vi "ysi.vi"(7 "Initialize":bool, 10 "Time Out (secs)":i32, 11 "YSI Com Port":i32) -> (0 "pH":dbl format="%.2f", 1 "Temperature":dbl format="%.2f", 2 "dis O2":dbl format="%.2f", 3 "ORP":dbl format="%.2f", 4 "spec K":dbl format="%.2f", 5 "Fresh Data":bool, 6 "Time out occurred":bool)   [LabVIEW 2016]
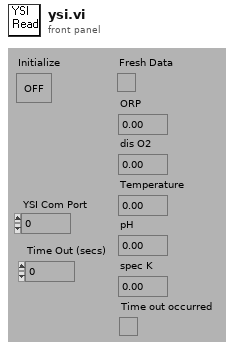
[diagram p1: front panel]
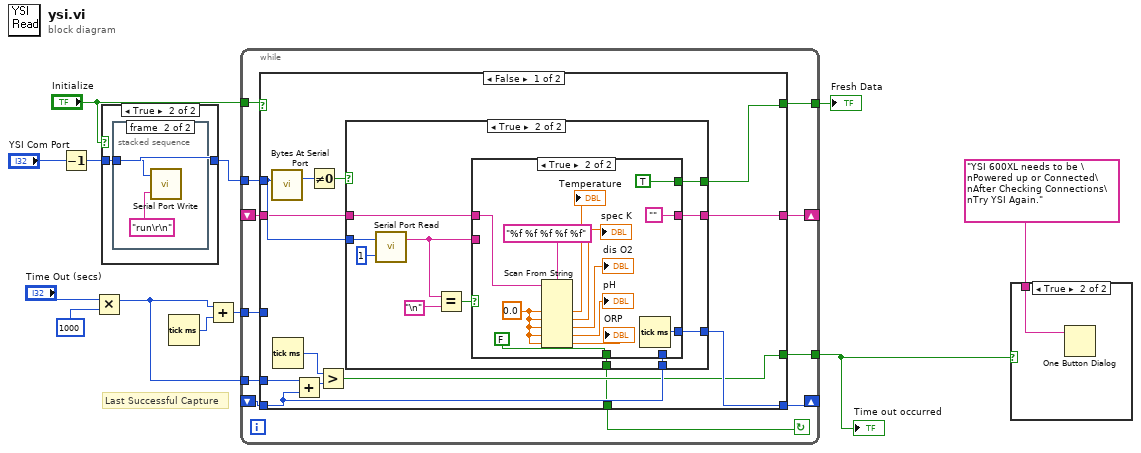
[diagram p0: block diagram]
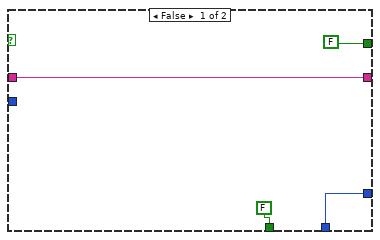
[diagram p2: hidden frame]
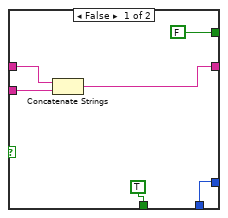
[diagram p3: hidden frame]
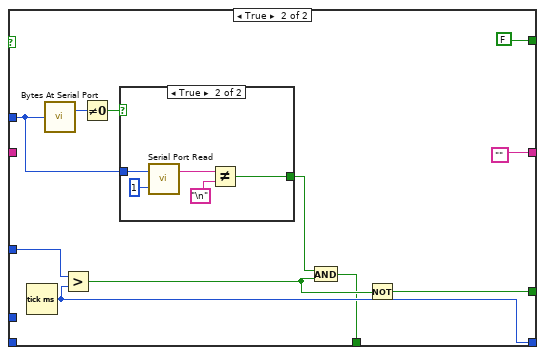
[diagram p4: hidden frame]
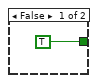
[diagram p5: hidden frame]
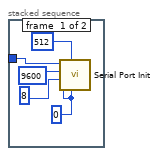
[diagram p8: hidden frame]
diagram:
  # "Last Successful Capture"
  n1 = Decrement(x="YSI Com Port") -> (x-1=w4:i32)
  n2 = Multiply(x="Time Out (secs)", y=1000) -> (x*y=w1:i32)
  n3 = case shown="True" "Initialize" {
    tunnel: w4 -> [w13 w14]
    tunnel: [w13 w14] -> w8
    frame False {
    }
    frame True {
      n4 = stacked-sequence {
        tunnel: w14 -> [w15 w21]
        frame #0 {
          w16 = 0
          n5 = call <vilib>:"Serial Port Init.vi"("parity"=w16, "buffer size"=512, "stop bits"=w16, "data bits"=8, "baud rate"=9600, "port number"=w15) -> ()  [unwired: 1 in, 1 out]
        }
        frame #1 {
          n6 = call <vilib>:"Serial Port Write.vi"("string to write"="run\r\n", "port number"=w21) -> ()  [unwired: 1 out]
        }
      }
    }
  }
  n7 = Tick Count (ms)() -> (millisecond timer value=w12:u32)
  n8 = Add(x=w1, y=w12) -> (x+y=w11:u32)
  n9 = while {
    tunnel: w1 -> [w22]
    tunnel: [w26] -> w6
    tunnel: [w28] -> w5
    shift-left: _ -> [w23]
    shift-right: [w29] -> _
    tunnel: w11 -> [w30]
    tunnel: w8 -> [w31]
    tunnel: "Initialize" -> [w32]
    shift-left: _ -> [w25]
    shift-right: [w24] -> _
    stop <- w27 continue-if-true
    n10 = case shown="False" w32 {
      tunnel: w31 -> [w44 w88]
      tunnel: w30 -> [_ w87]
      tunnel: [w40 w84] -> w29
      tunnel: [w36 w82] -> w28
      tunnel: [w34 w81] -> w27
      tunnel: [w41 FALSE] -> w26
      tunnel: w25 -> [w43 _]
      tunnel: [w42 ""] -> w24
      tunnel: w23 -> [w39 _]
      tunnel: w22 -> [w33 _]
      frame False {
        n11 = call <vilib>:"Bytes At Serial Port.vi"("port number"=w44) -> ("byte count"=w45:u32)  [unwired: 1 out]
        n12 = Tick Count (ms)() -> (millisecond timer value=w37:u32)
        n13 = Add(x=w33, y=w39) -> (x+y=w38:u32)
        n14 = Not Equal To 0?(x=w45) -> (x != 0?=w35:bool)
        n15 = Greater?(x=w37, y=w38) -> (0:w36:bool)
        n16 = case shown="True" w35 {
          tunnel: [w49 w57] -> w42
          tunnel: w44 -> [_ w55]
          tunnel: w43 -> [w49 w54]
          tunnel: [FALSE w53] -> w41
          tunnel: [w47 w52] -> w40
          tunnel: w39 -> [w47 w51]
          tunnel: [FALSE w50] -> w34
          frame False {
          }
          frame True {
            n17 = call <vilib>:"Serial Port Read.vi"("requested byte count"=1, "port number"=w55) -> ("string read"=w56:string)  [unwired: 1 out]
            n18 = Equal?(x=w56, y="\n") -> (x = y?=w58:bool)
            n19 = case shown="True" w58 {
              tunnel: [w65 ""] -> w57
              tunnel: w56 -> [w66 _]
              tunnel: w54 -> [w64 w73]
              tunnel: [FALSE TRUE] -> w53
              tunnel: [w62 w74] -> w52
              tunnel: w51 -> [w62 _]
              tunnel: [TRUE FALSE] -> w50
              frame False {
                n20 = Concatenate Strings(w64, w66) -> (w65:string)
              }
              frame True {
                w77 = 0.0
                n21 = Scan From String(format string="%f %f %f %f %f", input string=w73, default 1=w77, default 2=w77, default 3=w77, default 4=w77, default 5=w77) -> (output 1=→"Temperature":dbl, output 2=→"spec K":dbl, output 3=→"dis O2":dbl, output 4=→"pH":dbl, output 5=→"ORP":dbl)  [unwired: 2 in, 3 out]
                n22 = Tick Count (ms)() -> (millisecond timer value=w74:u32)
              }
            }
          }
        }
      }
      frame True {
        n23 = Tick Count (ms)() -> (millisecond timer value=w84:u32)
        n24 = call <vilib>:"Bytes At Serial Port.vi"("port number"=w88) -> ("byte count"=w89:u32)  [unwired: 1 out]
        n25 = Greater?(x=w87, y=w84) -> (0:w83:bool)
        n26 = Not Equal To 0?(x=w89) -> (x != 0?=w85:bool)
        n27 = case shown="True" w85 {
          tunnel: w88 -> [_ w92]
          tunnel: [TRUE w91] -> w86
          frame False {
          }
          frame True {
            n28 = call <vilib>:"Serial Port Read.vi"("requested byte count"=1, "port number"=w92) -> ("string read"=w93:string)  [unwired: 1 out]
            n29 = Not Equal?(x=w93, y="\n") -> (x != y?=w91:bool)
          }
        }
        n30 = And(x=w86, y=w83) -> (x .and. y?=w81:bool)
        n31 = Not(x=w83) -> (.not. x?=w82:bool)
      }
    }
  }
  "Fresh Data" <- w6
  "Time out occurred" <- w5
  n32 = case shown="True" w5 {
    tunnel: "YSI 600XL needs to be \nPowered up or Connected\nAfter Checking Connections\nTry YSI Again." -> [_ w96]
    frame False {
    }
    frame True {
      n33 = One Button Dialog(message=w96) -> ()  [unwired: 1 in, 1 out]
    }
  }
